vi "Create Tag Path.vi"(9 "channel name":string, 10 "group name":string) -> (3 "tag path":string)   [LabVIEW 2020, in "FlexLoggerTagHelpers.lvlib"]
uses:
  FlexLoggerTagHelpers.lvlib
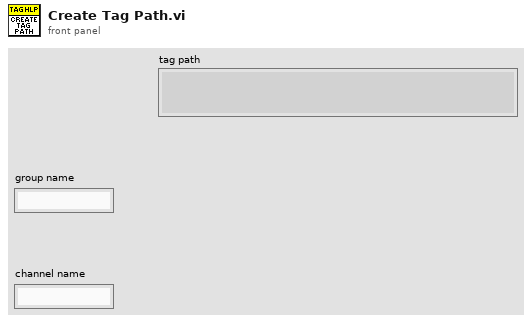
[diagram p1: front panel]
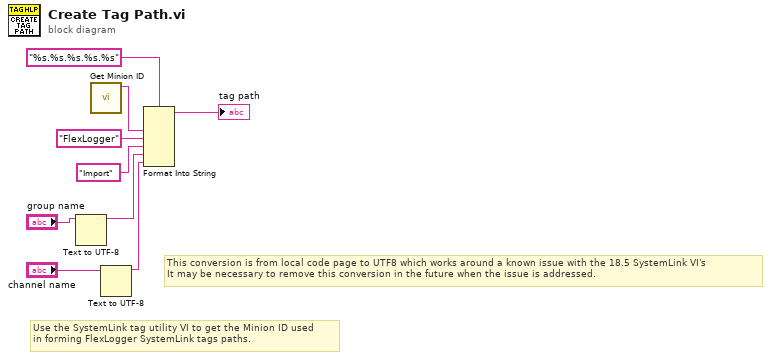
[diagram p0: block diagram]
diagram:
  # "This conversion is from local code page to UTF8 which works around a known issue with the 18.5 SystemLink VI's\nIt may be necessary to remove this conversion in the future when the issue is addressed."
  # "Use the SystemLink tag utility VI to get the Minion ID used\nin forming FlexLogger SystemLink tags paths."
  n1 = Text to UTF-8(11:"group name") -> (3:w3:string)  [unwired: 2 in, 1 out]
  n2 = call <vilib>:"Get Minion ID.vi"() -> ("minion id"=w8:string)  [unwired: 11 in]
  n3 = Text to UTF-8(11:"channel name") -> (3:w1:string)  [unwired: 2 in, 1 out]
  n4 = Format Into String(format string="%s.%s.%s.%s.%s", w8, "FlexLogger" ("string"), "Import" ("string"), w3, w1) -> (resulting string=→"tag path":string)  [unwired: 2 in, 1 out]
